vi "multi_pub.vi"() -> ()   [LabVIEW 2022 SP3]
uses:
  D:/UOM/EE2044 - Electrical Measurements and Instrumentation/Project/Measurment Project/Quaxo_MQTT_LabVIEW-master/Controls/QoS.ctl
  D:/UOM/EE2044 - Electrical Measurements and Instrumentation/Project/Measurment Project/Quaxo_MQTT_LabVIEW-master/Controls/Retain_Flag.ctl
  D:/UOM/EE2044 - Electrical Measurements and Instrumentation/Project/Measurment Project/Quaxo_MQTT_LabVIEW-master/Controls/DUP_Flag.ctl
  D:/UOM/EE2044 - Electrical Measurements and Instrumentation/Project/Measurment Project/Quaxo_MQTT_LabVIEW-master/Controls/Connection_Return_Codes.ctl
  D:/UOM/EE2044 - Electrical Measurements and Instrumentation/Project/Measurment Project/Quaxo_MQTT_LabVIEW-master/Controls/Connect_Flags.ctl
  D:/UOM/EE2044 - Electrical Measurements and Instrumentation/Project/Measurment Project/Quaxo_MQTT_LabVIEW-master/Controls/User_Info.ctl
  D:/UOM/EE2044 - Electrical Measurements and Instrumentation/Project/Measurment Project/Quaxo_MQTT_LabVIEW-master/MQTT_Functions.lvlib
panel:
  in  "Topic 3":string="testtopic/Node12345"
  in  "Message to be published 3":string="Quaxo says it's "
  in  "Message to be published 2":string="Quaxo says it's "
  in  "Topic 2":string="testtopic/Node12345"
  out "Connection Status":T1=enum."Connection refused: not authorized"
  in  "Stop Publishing":bool
  out "Message published":string
  in  "MQTT Broker":cluster{"address (IP)":string, "port":u16}={"address (IP)"="broker.mqttdashboard.com", "port"=1883}
  in  "Message to be published1":string="Quaxo says it's "
  in  "Client ID":string="NodeE-12345"
  in  "Topic1":string="testtopic/Node12345"
  in  "Publish Meta":cluster{"QoS":T2, "Retain":T3, "DUP":T4}
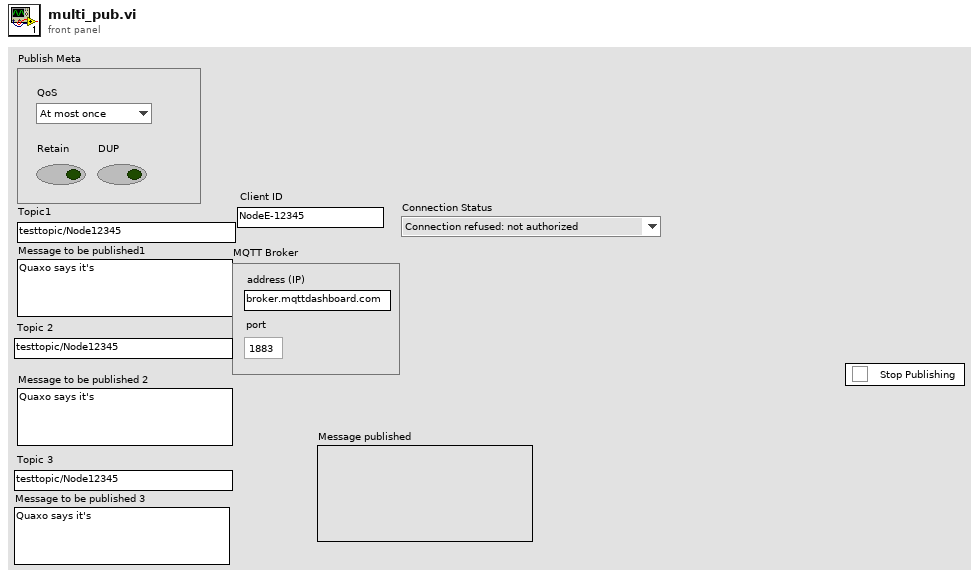
[diagram p1: front panel]
types:
  T1 = typedef "MQTT_Functions.lvlib/Connection_Return_Codes.ctl" = enum16{"Connection accepted", "Connection refused: unacceptable protocol version", "Connection refused: identifier rejected", "Connection refused: Server unavailable", "Connection refused: bad user name or password", "Connection refused: not authorized"}
  T2 = typedef "MQTT_Functions.lvlib/QoS.ctl" = enum8{"At most once", "At least once", "Exactly once", "Reserved"}
  T3 = typedef "MQTT_Functions.lvlib/Retain_Flag.ctl" = bool
  T4 = typedef "MQTT_Functions.lvlib/DUP_Flag.ctl" = bool
  T5 = typedef "MQTT_Functions.lvlib/User_Info.ctl" = cluster{"User Name":string, "Password":string}
  T6 = typedef "MQTT_Functions.lvlib/Connect_Flags.ctl" = cluster{"user name":bool, "password":bool, "will retain":bool, "will flag":bool, "clean session":bool, "reserved":bool, "will QoS":T2}
  T7 = cluster{"QoS":T2, "DUP":T4, "Retain":T3, "Keep Alive (sec)":u16}
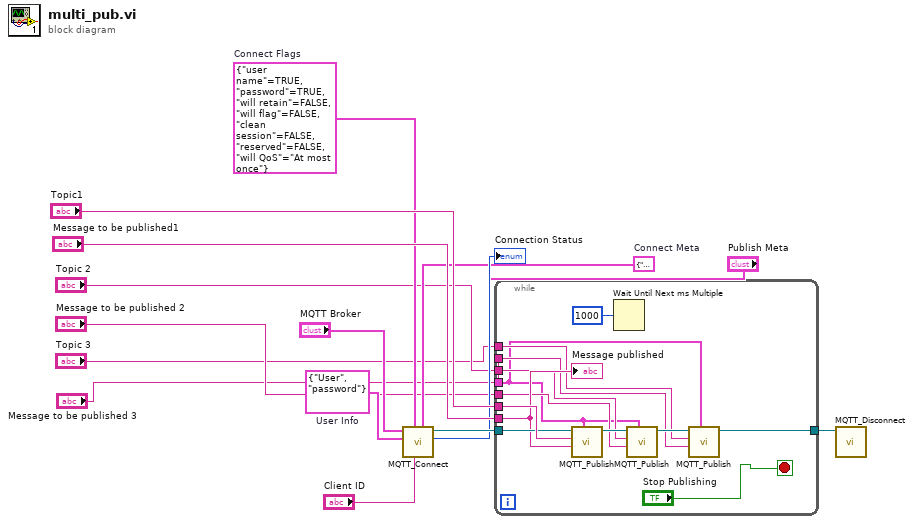
[diagram p0: block diagram]
diagram:
  w7 = T5 {"User Name"="User", "Password"="password"}  # User Info
  w13 = T6 {"user name"=TRUE, "password"=TRUE, "will retain"=FALSE, "will flag"=FALSE, "clean session"=FALSE, "reserved"=FALSE, "will QoS"=enum."At most once"}  # Connect Flags
  w6 = T7 {"QoS"=enum."At most once", "DUP"=FALSE, "Retain"=FALSE, "Keep Alive (sec)"=60}  # Connect Meta
  n1 = call "MQTT_Connect.vi"("Connect Meta"=w6, "Client ID"="Client ID", "Connect Flags"=w13, "User Info"=w7, "MQTT Broker"="MQTT Broker") -> ("Connection Status"=→"Connection Status":T1, "connection ID out"=w9:refnum<k5>)  [unwired: 4 in, 1 out]
  n2 = while {
    tunnel: "Topic1" -> [w28]
    tunnel: "Message to be published1" -> [w25]
    tunnel: w9 -> [w27]
    tunnel: [w20] -> w11
    tunnel: "Topic 2" -> [w23]
    tunnel: "Message to be published 2" -> [w22]
    tunnel: "Topic 3" -> [w19]
    tunnel: "Message to be published 3" -> [w18]
    tunnel: "Publish Meta" -> [w17]
    stop <- "Stop Publishing" stop-if-true
    n3 = call "MQTT_Publish.vi"("Publish Meta"=w17, "Message to be published"=w25, "Topic"=w28, "connection ID"=w27) -> ("connection ID out"=w24:refnum<k5>)  [unwired: 6 in, 1 out]
    n4 = Wait Until Next ms Multiple(millisecond multiple=u32 1000) -> ()  [unwired: 1 out]
    n5 = call "MQTT_Publish.vi"("Publish Meta"=w17, "Message to be published"=w22, "Topic"=w23, "connection ID"=w24) -> ("connection ID out"=w21:refnum<k5>)  [unwired: 6 in, 1 out]
    n6 = call "MQTT_Publish.vi"("Publish Meta"=w17, "Message to be published"=w18, "Topic"=w19, "connection ID"=w21) -> ("connection ID out"=w20:refnum<k5>)  [unwired: 6 in, 1 out]
    "Message published" <- w25
  }
  n7 = call "MQTT_Disconnect.vi"("connection ID"=w11) -> ()  [unwired: 10 in, 1 out]
